vi "JSONRPC-ArrayIsEmpty.vi"(11 "input array":string[](array[string])=["intout", "stringout", "time"]) -> (3 "empty?":bool)   [LabVIEW 2015]
doc: "empty? is true if and only if <b>input array</b> has length<0 or only one element and contains an empty string."
panel:
  # "ArrayIsEmpty"
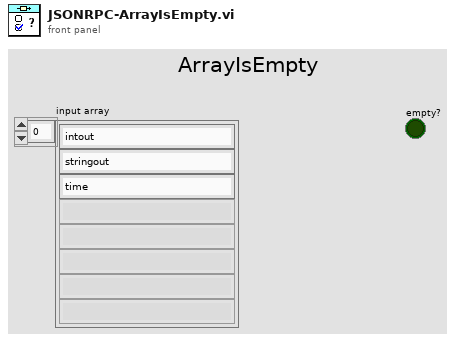
[diagram p1: front panel]
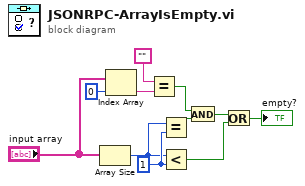
[diagram p0: block diagram]
diagram:
  w3 = 1 ("y")
  n1 = Array Size(array="input array") -> (size(s)=w2:i32)
  n2 = Index Array(array="input array", index=0) -> (element=w10:string)
  n3 = Equal?(x="", y=w10) -> (x = y?=w7:bool)
  n4 = Equal?(x=w2, y=w3) -> (x = y?=w5:bool)
  n5 = Less?(x=w2, y=w3) -> (x < y?=w1:bool)
  n6 = And(x=w7, y=w5) -> (x .and. y?=w4:bool)
  n7 = Or(x=w4, y=w1) -> (x .or. y?=→"empty?":bool)
